vi "trigger-test3.vi"() -> ()   [LabVIEW 2020]
uses:
  Realization/PI650 VoltageAmp/TypeDefs/Channel gain.ctl
  Realization/PIPX40 Matrix/PIPX40 Matrix.lvclass
  Realization/PI650 VoltageAmp/PI650 VoltageAmp.lvclass
  Realization/PI650 VoltageAmp/TypeDefs/Channel DC offset.ctl
  Realization/NI PXI Trigger/NI PXI Trigger.lvclass
  Realization/NI PXI Trigger/PXI Trigger config.ctl
  Realization/NI DMM/NI DMM.lvclass
  Realization/NI DMM/TypeDefs/DMM waveform settings.ctl
  <instrlib>/niDMM/nidmm.llb/niDMM Waveform Function.ctl
  Realization/NI DMM/TypeDefs/Trigger settings.ctl
  <instrlib>/niDMM/nidmm.llb/niDMM Trigger.ctl
  <instrlib>/niDMM/nidmm.llb/niDMM Slope.ctl
  Realization/NI Analog Input/NI Analog Input.lvclass
  Realization/NI DAQmx Base/TypeDefs/Channel Config.ctl
  Realization/NI Analog Output/TypeDefs/Trigger Config.ctl
  Realization/NI Analog Output/NI Analog Output.lvclass
  Realization/NI Analog Output/TypeDefs/Timing Config.ctl
  <vilib>/measure/NI_MABase.lvlib
panel:
  in  "noise level":dbl=0.05 format="%#_3f"
  in  "signal type":T1(ring)
  in  "Channel gain":T2={"Channel (CH1)"=3, "Gain (x1)"=2} {"Channel (CH1)" items=["CH1"=1, "CH2"=2, "CH3"=3, "CH4"=4, "CH5"=5]; "Gain (x1)" items=["x1"=1, "x2"=2, "x5"=3, "x7"=4, "x10"=5, "x14"=6, "x20"=7]}
  out "Amp Info":variant
  out "Mx infos":variant[](array[variant])
  out "Waveform Graph":dynamicdata(graph)
  out "error out":errorcluster
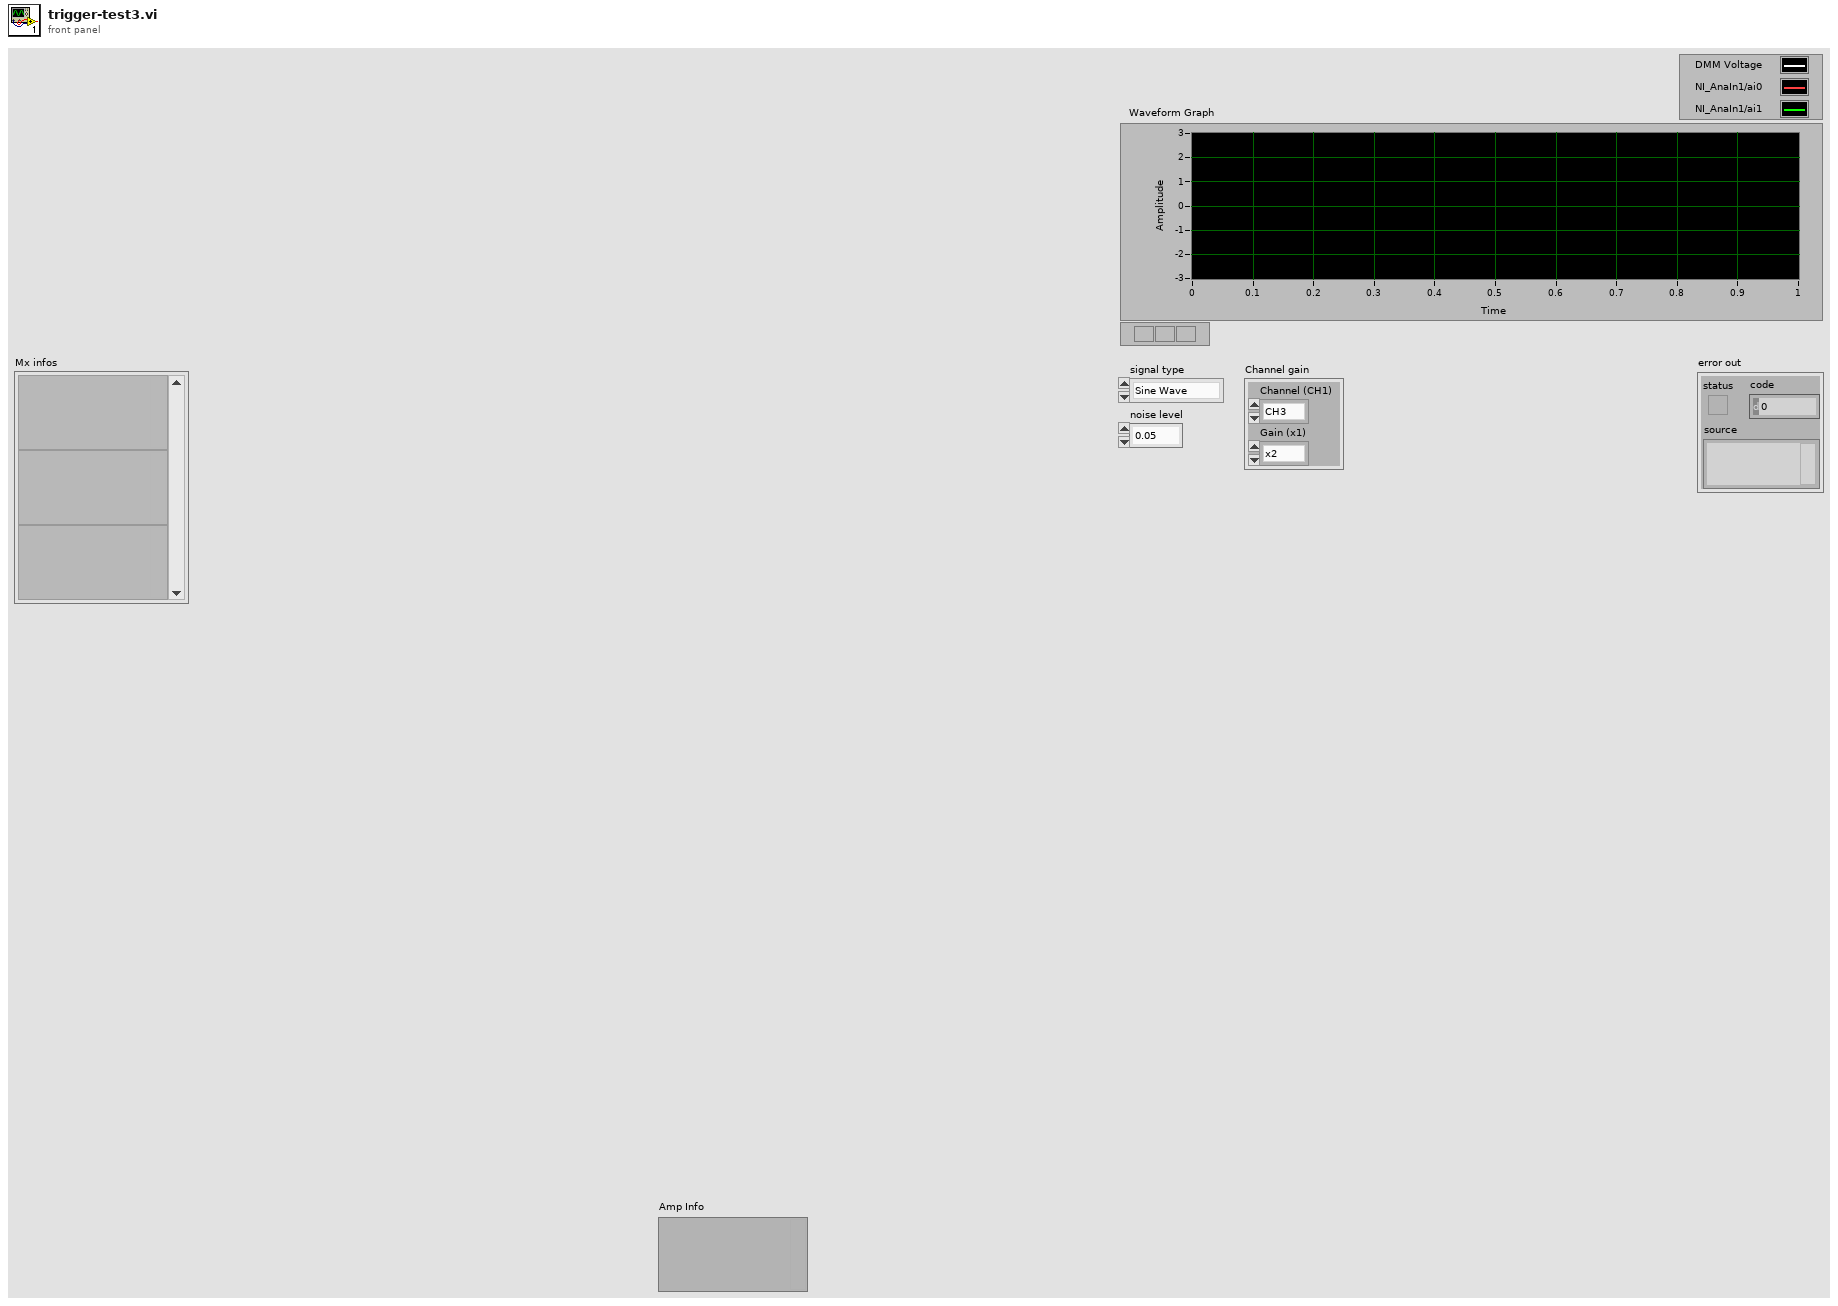
[diagram p1: front panel]
types:
  T1 = enum16{"Sine Wave", "Triangle Wave", "Square Wave", "Sawtooth Wave"}
  T2 = typedef "Channel gain.ctl" = cluster{"Channel (CH1)":u32, "Gain (x1)":u32}
  T3 = typedef "Trigger Config.ctl" = cluster{"trigger type":string, "source":string, "slope":i32, "analog level":dbl, "analog hysteresis":dbl}
  T4 = typedef "Timing Config.ctl" = cluster{"sample mode":i32, "samples per channel":i32, "rate":dbl, "source":string, "active edge":i32}
  T5 = typedef "Channel Config.ctl" = cluster{"channels":string, "maximum value":dbl, "minimum value":dbl, "output terminal configuration":i32, "units":i32}
  T6 = typedef "Trigger settings.ctl" = cluster{"Trigger Source":T7, "Trigger Delay (sec)":dbl, "Slope":T8}
  T7 = typedef "niDMM Trigger.ctl" = enum16{"Immediate", "External", "TTL 0", "TTL 1", "TTL 2", "TTL 3", "TTL 4", "TTL 5", "TTL 6", "Software", "TTL 7", "PXI Star", "LBR Trig 1", "Aux Trig 1"}
  T8 = typedef "niDMM Slope.ctl" = enum16{"Rising Edge", "Falling Edge"}
  T9 = typedef "DMM waveform settings.ctl" = cluster{"Waveform Points":i32, "Function":T10, "Rate":dbl, "Range":dbl, "\nSettle Time":dbl}
  T10 = typedef "niDMM Waveform Function.ctl" = i32
  T11 = typedef "PXI Trigger config.ctl" = cluster{"counter output":string, "source terminal":string, "destination terminal":string}
  T12 = typedef "Channel DC offset.ctl" = cluster{"Channel (CH1)":u32, "Offset (128)":u32}
  T13 = map{string, refnum<class "PIPX40 Matrix.lvclass">}
  T14 = cluster{"samples per channel":dbl, "samples per channel":dbl}
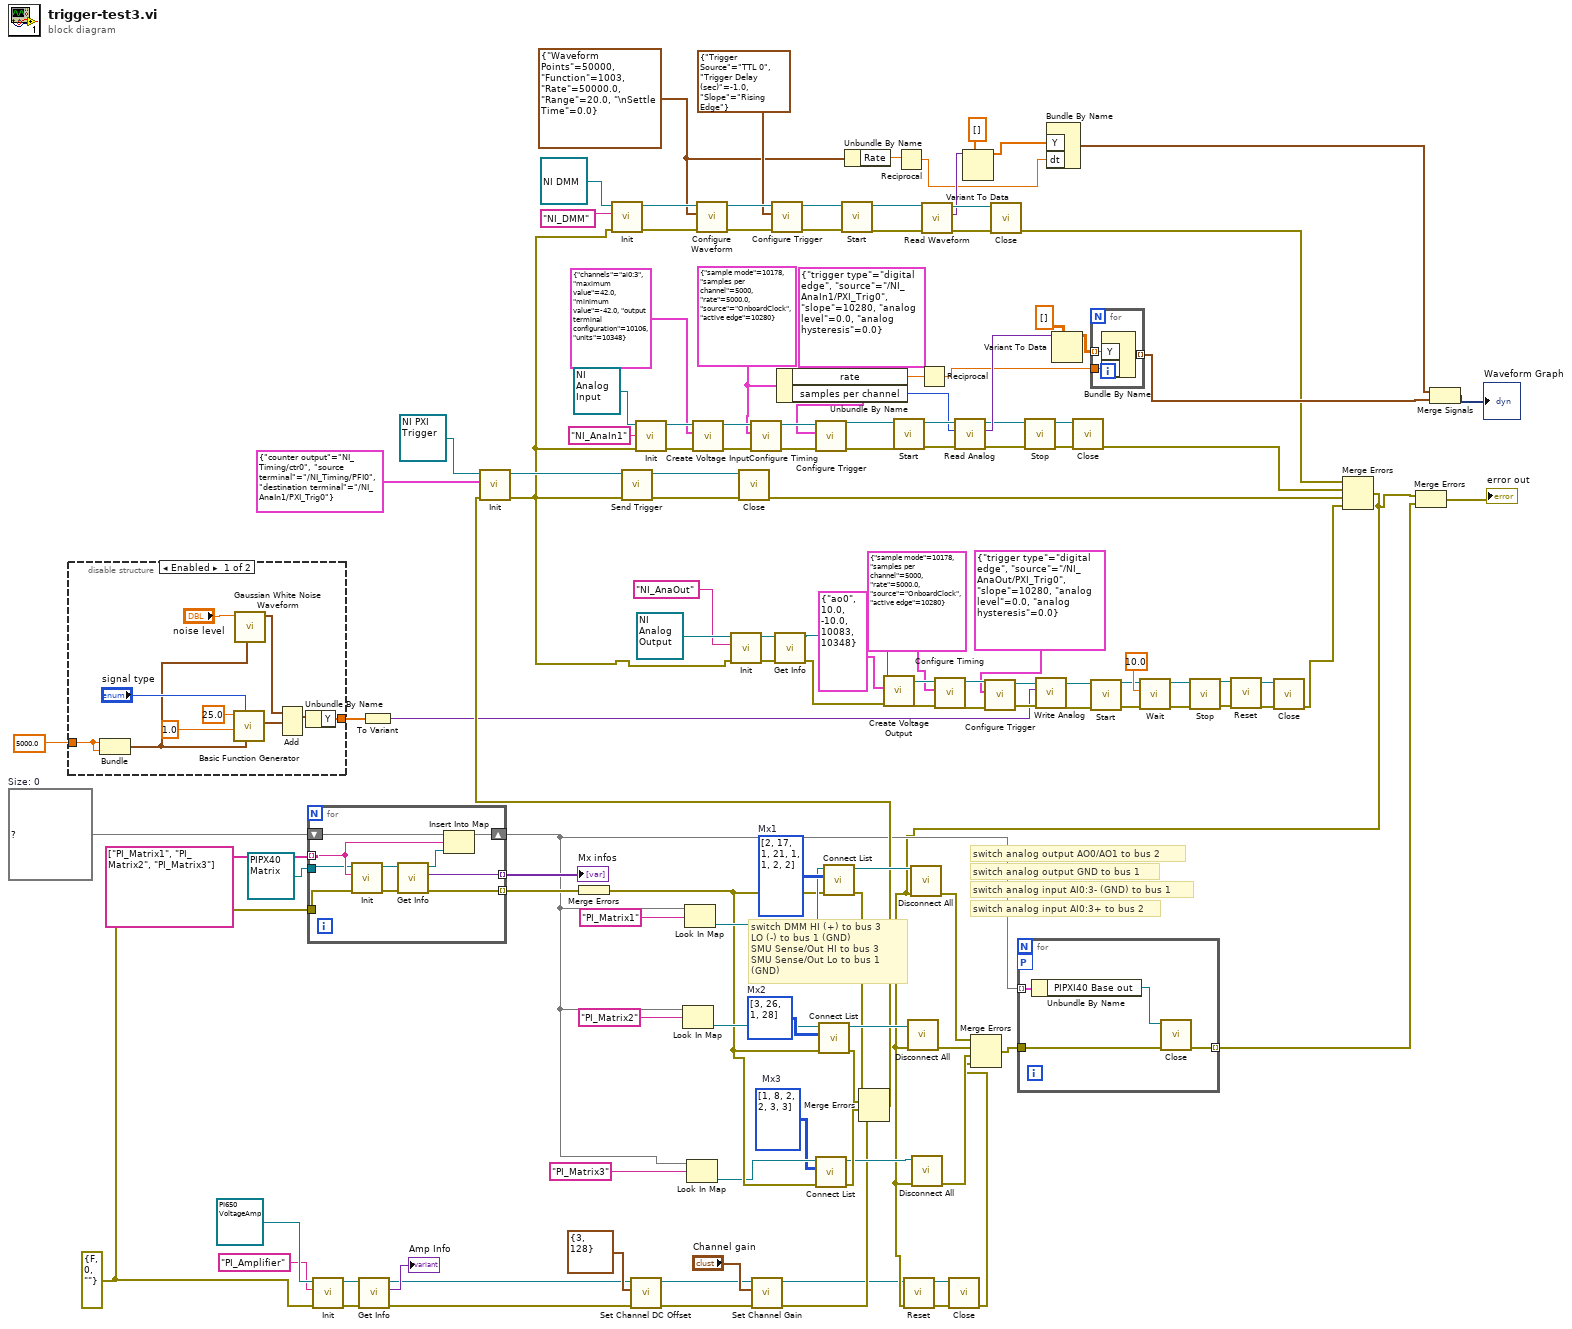
[diagram p0: block diagram]
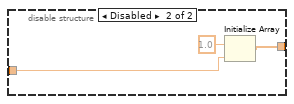
[diagram p2: hidden frame]
diagram:
  w32 = T4 {"sample mode"=10178, "samples per channel"=5000, "rate"=5000.0, "source"="OnboardClock", "active edge"=10280}
  w60 = T9 {"Waveform Points"=50000, "Function"=1003, "Rate"=50000.0, "Range"=20.0, "\nSettle Time"=0.0}
  w94 = errorcluster {"status"=FALSE, "code"=0, "source"=""} ("error in (no error)")
  w105 = i32[][] [[1, 8], [2, 2], [3, 3]]  # Mx3
  w116 = T13 {}  # Size: 0
  w125 = i32[][] [[3, 26], [1, 28]]  # Mx2
  w127 = i32[][] [[2, 17], [1, 21], [1, 1], [2, 2]]  # Mx1
  # "switch analog input AI0:3+ to bus 2"
  # "switch analog input AI0:3- (GND) to bus 1"
  # "switch analog output GND to bus 1"
  # "switch analog output AO0/AO1 to bus 2"
  # "switch DMM HI (+) to bus 3 \nLO (-) to bus 1 (GND)\nSMU Sense/Out HI to bus 3\nSMU Sense/Out Lo to bus 1 (GND)"
  n1 = disable-structure shown="Enabled" {
    disable-tunnel: 5000.0 ("samples per channel") -> [w141 w144]
    disable-tunnel: [w140 w146] -> w83
    frame Enabled {
      n2 = Bundle("samples per channel"=w141, "samples per channel"=w141) -> (w138:T14)  [unwired: 1 in]
      n3 = call <vilib>:"Basic Function Generator.vi"("sampling info"=w138, "signal type"="signal type", "amplitude"=1.0, "frequency"=25.0) -> ("signal out"=w137:waveform(dbl))  [unwired: 5 in, 2 out]
      n4 = call <vilib>:"Gaussian White Noise Waveform.vi"("sampling info"=w138, "standard deviation"="noise level") -> ("signal out"=w136:waveform(dbl))  [unwired: 8 in, 1 out]
      n5 = Add(1:w137, 2:w136) -> (0:w135:waveform(dbl))  [unwired: 1 in, 1 out]
      n6 = Unbundle By Name(w135) -> ("Y"=w140:dbl[])
    }
    frame Disabled {
      n7 = Initialize Array(1.0 ("element"), w144) -> (w146:dbl[])
    }
  }
  n8 = for {
    tunnel: string[] ["PI_Matrix1", "PI_Matrix2", "PI_Matrix3"] -> [w152] mode=indexing
    tunnel: [w155] -> w130 mode=indexing
    tunnel: [w154] -> w129 mode=indexing
    shift-right: [w153] -> w108
    shift-left: w116 -> [w150]
    tunnel: refnum<class "PIPX40 Matrix.lvclass"> refnum ("PIPXI40 Matrix in") -> [w148]
    tunnel: w94 -> [w147]
    n9 = call-dynamic "Init.vi"("error in (no error)"=w147, "Params"=w152, "PIPXI40 Base in"=w148) -> ("error out"=w156:errorcluster, "PIPXI40 Base out"=w151:refnum<class "PIPX40 Matrix.lvclass">)  [unwired: 7 in]
    n10 = call-dynamic "Get Info.vi"("error in (no error)"=w156, "PIPXI40 Base in"=w151) -> ("error out"=w155:errorcluster, "Info"=w154:variant, "PIPXI40 Base out"=w149:refnum<class "PIPX40 Matrix.lvclass">)  [unwired: 7 in]
    n11 = Insert Into Map(map in=w150, key=w152, value=w149) -> (map out=w153:T13)  [unwired: 2 out]
  }
  "Mx infos" <- w129
  n12 = call-dynamic "Init.vi"("error in (no error)"=w94, "Params"="PI_Amplifier" ("String"), "PI650 VoltageAmp in"=refnum<class "PI650 VoltageAmp.lvclass"> refnum) -> ("error out"=w99:errorcluster, "PI650 VoltageAmp out"=w100:refnum<class "PI650 VoltageAmp.lvclass">)  [unwired: 7 in]
  n13 = call-dynamic "Get Info.vi"("error in (no error)"=w99, "PI650 VoltageAmp in"=w100) -> ("error out"=w93:errorcluster, "Info"=→"Amp Info":variant, "PI650 VoltageAmp out"=w92:refnum<class "PI650 VoltageAmp.lvclass">)  [unwired: 7 in]
  n14 = To Variant(anything=w83) -> (Variant=w1:variant)
  n15 = Merge Errors(w130) -> (w107:errorcluster)
  n16 = call-dynamic "Set Channel DC Offset.vi"("error in (no error)"=w93, "Params"=T12 {"Channel (CH1)"=3, "Offset (128)"=128}, "PI650 VoltageAmp in"=w92) -> ("error out"=w90:errorcluster, "PI650 VoltageAmp out"=w91:refnum<class "PI650 VoltageAmp.lvclass">)  [unwired: 7 in]
  n17 = Look In Map(map=w108, key="PI_Matrix2" ("String")) -> (value=w118:refnum<class "PIPX40 Matrix.lvclass">)  [unwired: 1 in, 1 out]
  n18 = Look In Map(map=w108, key="PI_Matrix1" ("String")) -> (value=w119:refnum<class "PIPX40 Matrix.lvclass">)  [unwired: 1 in, 1 out]
  n19 = Look In Map(map=w108, key="PI_Matrix3" ("String")) -> (value=w106:refnum<class "PIPX40 Matrix.lvclass">)  [unwired: 1 in, 1 out]
  n20 = call-dynamic "Set Channel Gain.vi"("error in (no error)"=w90, "Params"="Channel gain", "PI650 VoltageAmp in"=w91) -> ("error out"=w89:errorcluster, "PI650 VoltageAmp out"=w85:refnum<class "PI650 VoltageAmp.lvclass">)  [unwired: 7 in]
  n21 = Unbundle By Name(w32) -> ("rate"=w30:dbl, "samples per channel"=w31:i32)
  n22 = call-dynamic "Connect List.vi"("error in (no error)"=w107, "Params"=w105, "PIPXI40 Matrix in"=w106) -> ("error out"=w104:errorcluster, "PIPXI40 Matrix out"=w103:refnum<class "PIPX40 Matrix.lvclass">)  [unwired: 7 in]
  n23 = call-dynamic "Connect List.vi"("error in (no error)"=w107, "Params"=w125, "PIPXI40 Matrix in"=w118) -> ("error out"=w114:errorcluster, "PIPXI40 Matrix out"=w123:refnum<class "PIPX40 Matrix.lvclass">)  [unwired: 7 in]
  n24 = call-dynamic "Connect List.vi"("error in (no error)"=w107, "Params"=w127, "PIPXI40 Matrix in"=w119) -> ("error out"=w115:errorcluster, "PIPXI40 Matrix out"=w124:refnum<class "PIPX40 Matrix.lvclass">)  [unwired: 7 in]
  n25 = Unbundle By Name(w60) -> ("Rate"=w59:dbl)
  n26 = Merge Errors(w115, w114, w104, w89) -> (w113:errorcluster)
  n27 = call-dynamic "Init.vi"("error in (no error)"=w113, "Params"=T11 {"counter output"="NI_Timing/ctr0", "source terminal"="/NI_Timing/PFI0", "destination terminal"="/NI_AnaIn1/PXI_Trig0"} ("Cluster of class private data"), "NI PXI Trigger in"=refnum<class "NI PXI Trigger.lvclass"> refnum) -> ("error out"=w2:errorcluster, "NI PXI Trigger out"=w80:refnum<class "NI PXI Trigger.lvclass">)  [unwired: 7 in]
  n28 = call-dynamic "Init.vi"("error in (no error)"=w2, "Params"="NI_DMM", "NI DMM in"=refnum<class "NI DMM.lvclass"> refnum) -> ("error out"=w75:errorcluster, "NI DMM out"=w76:refnum<class "NI DMM.lvclass">)  [unwired: 7 in]
  n29 = call-dynamic "Send Trigger.vi"("error in (no error)"=w2, "NI PXI Trigger in"=w80) -> ("error out"=w79:errorcluster, "NI PXI Trigger out"=w78:refnum<class "NI PXI Trigger.lvclass">)  [unwired: 8 in]
  n30 = call-dynamic "Init.vi"("error in (no error)"=w2, "Params"="NI_AnaIn1" ("String"), "DAQmx Base in"=refnum<class "NI Analog Input.lvclass"> refnum ("NI Analog Input in")) -> ("error out"=w52:errorcluster, "DAQmx Base out"=w51:refnum<class "NI Analog Input.lvclass">)  [unwired: 7 in]
  n31 = call-dynamic "Create Voltage Input.vi"("error in (no error)"=w52, "Params"=T5 {"channels"="ai0:3", "maximum value"=42.0, "minimum value"=-42.0, "output terminal configuration"=10106, "units"=10348} ("Channel Config"), "NI Analog Input in"=w51) -> ("error out"=w53:errorcluster, "NI Analog Input out"=w50:refnum<class "NI Analog Input.lvclass">)  [unwired: 7 in]
  n32 = call-dynamic "Configure Waveform.vi"("error in (no error)"=w75, "Params"=w60, "NI DMM in"=w76) -> ("error out"=w71:errorcluster, "NI DMM out"=w72:refnum<class "NI DMM.lvclass">)  [unwired: 7 in]
  n33 = call-dynamic "Init.vi"("error in (no error)"=w2, "Params"="NI_AnaOut" ("String"), "DAQmx Base in"=refnum<class "NI Analog Output.lvclass"> refnum ("NI DAQmx.lvlib:NI Analog Output.lvclass")) -> ("error out"=w26:errorcluster, "DAQmx Base out"=w27:refnum<class "NI Analog Output.lvclass">)  [unwired: 7 in]
  n34 = call-dynamic "Close.vi"("error in (no error)"=w79, "NI PXI Trigger in"=w78) -> ("error out"=w56:errorcluster)  [unwired: 8 in, 1 out]
  n35 = call-dynamic "Configure Timing.vi"("error in (no error)"=w53, "Params"=w32, "NI DAQmx Base in"=w50) -> ("error out"=w48:errorcluster, "NI DAQmx Base out"=w49:refnum<class "NI Analog Input.lvclass">)  [unwired: 7 in]
  n36 = call-dynamic "Configure Trigger.vi"("error in (no error)"=w71, "Params"=T6 {"Trigger Source"=enum."TTL 0", "Trigger Delay (sec)"=-1.0, "Slope"=enum."Rising Edge"}, "NI DMM in"=w72) -> ("error out"=w69:errorcluster, "NI DMM out"=w70:refnum<class "NI DMM.lvclass">)  [unwired: 7 in]
  n37 = call-dynamic "Get Info.vi"("error in (no error)"=w26, "DAQmx Base in"=w27) -> ("error out"=w3:errorcluster, "DAQmx Base out"=w23:refnum<class "NI Analog Output.lvclass">)  [unwired: 7 in, 1 out]
  n38 = call-dynamic "Configure Trigger.vi"("error in (no error)"=w48, "Params"=T3 {"trigger type"="digital edge", "source"="/NI_AnaIn1/PXI_Trig0", "slope"=10280, "analog level"=0.0, "analog hysteresis"=0.0}, "NI DAQmx Base in"=w49) -> ("error out"=w42:errorcluster, "NI DAQmx Base out"=w41:refnum<class "NI Analog Input.lvclass">)  [unwired: 7 in]
  n39 = call-dynamic "Start.vi"("error in (no error)"=w69, "DMM in"=w70) -> ("error out"=w67:errorcluster, "DMM out"=w68:refnum<class "NI DMM.lvclass">)  [unwired: 8 in]
  n40 = call-dynamic "Create Voltage Output.vi"("error in (no error)"=w3, "Params"=T5 {"channels"="ao0", "maximum value"=10.0, "minimum value"=-10.0, "output terminal configuration"=10083, "units"=10348} ("Channel Config"), "NI Analog Output in"=w23) -> ("error out"=w22:errorcluster, "NI Analog Output out"=w21:refnum<class "NI Analog Output.lvclass">)  [unwired: 7 in]
  n41 = call-dynamic "Start.vi"("error in (no error)"=w42, "NI DAQmx Base in"=w41) -> ("error out"=w43:errorcluster, "NI DAQmx Base out"=w40:refnum<class "NI Analog Input.lvclass">)  [unwired: 8 in]
  n42 = Reciprocal(x=w59) -> (1/x=w58:dbl)
  n43 = Reciprocal(x=w30) -> (1/x=w29:dbl)
  n44 = call-dynamic "Read Waveform.vi"("error in (no error)"=w67, "NI DMM in"=w68) -> ("error out"=w65:errorcluster, "Data"=w63:variant, "NI DMM out"=w64:refnum<class "NI DMM.lvclass">)  [unwired: 7 in]
  n45 = call-dynamic "Configure Timing.vi"("error in (no error)"=w22, "Params"=T4 {"sample mode"=10178, "samples per channel"=5000, "rate"=5000.0, "source"="OnboardClock", "active edge"=10280}, "NI DAQmx Base in"=w21) -> ("error out"=w8:errorcluster, "NI DAQmx Base out"=w7:refnum<class "NI Analog Output.lvclass">)  [unwired: 7 in]
  n46 = call-dynamic "Read Analog.vi"("error in (no error)"=w43, "Params"=w31, "NI Analog Input in"=w40) -> ("error out"=w35:errorcluster, "Data"=w38:variant, "NI Analog Input out"=w36:refnum<class "NI Analog Input.lvclass">)  [unwired: 6 in]
  n47 = Variant To Data(type=dbl[] [], Variant=w63) -> (data=w61:dbl[])  [unwired: 1 in, 1 out]
  n48 = call-dynamic "Configure Trigger.vi"("error in (no error)"=w8, "Params"=T3 {"trigger type"="digital edge", "source"="/NI_AnaOut/PXI_Trig0", "slope"=10280, "analog level"=0.0, "analog hysteresis"=0.0}, "NI DAQmx Base in"=w7) -> ("error out"=w5:errorcluster, "NI DAQmx Base out"=w6:refnum<class "NI Analog Output.lvclass">)  [unwired: 7 in]
  n49 = call-dynamic "Close.vi"("error in (no error)"=w65, "NI DMM in"=w64) -> ("error out"=w54:errorcluster)  [unwired: 8 in, 1 out]
  n50 = call-dynamic "Stop.vi"("error in (no error)"=w35, "NI DAQmx Base in"=w36) -> ("error out"=w34:errorcluster, "NI DAQmx Base out"=w37:refnum<class "NI Analog Input.lvclass">)  [unwired: 8 in]
  n51 = call-dynamic "Write Analog.vi"("error in (no error)"=w5, "Params"=w1, "NI Analog Output in"=w6) -> ("error out"=w19:errorcluster, "NI Analog Output out"=w18:refnum<class "NI Analog Output.lvclass">)  [unwired: 7 in]
  n52 = Bundle By Name("Y"=w61, "dt"=w58) -> (w57:waveform(dbl))  [unwired: 1 in]
  n53 = Variant To Data(type=dbl[][] [], Variant=w38) -> (data=w33:dbl[][])  [unwired: 1 in, 1 out]
  n54 = call-dynamic "Close.vi"("error in (no error)"=w34, "DAQmx Base in"=w37) -> ("error out"=w55:errorcluster)  [unwired: 8 in, 1 out]
  n55 = for {
    tunnel: w33 -> [w159] mode=indexing
    tunnel: [w158] -> w82 mode=indexing
    tunnel: w29 -> [w157]
    n56 = Bundle By Name("Y"=w159, "dt"=w157) -> (w158:waveform(dbl))  [unwired: 1 in]
  }
  n57 = call-dynamic "Start.vi"("error in (no error)"=w19, "NI DAQmx Base in"=w18) -> ("error out"=w12:errorcluster, "NI DAQmx Base out"=w11:refnum<class "NI Analog Output.lvclass">)  [unwired: 8 in]
  n58 = call-dynamic "Wait.vi"("error in (no error)"=w12, "Params"=10.0, "NI DAQmx Base in"=w11) -> ("error out"=w14:errorcluster, "NI DAQmx Base out"=w15:refnum<class "NI Analog Output.lvclass">)  [unwired: 7 in]
  n59 = call-dynamic "Stop.vi"("error in (no error)"=w14, "NI DAQmx Base in"=w15) -> ("error out"=w17:errorcluster, "NI DAQmx Base out"=w16:refnum<class "NI Analog Output.lvclass">)  [unwired: 8 in]
  n60 = call-dynamic "Reset.vi"("error in (no error)"=w17, "DAQmx Base in"=w16) -> ("error out"=w10:errorcluster, "DAQmx Base out"=w9:refnum<class "NI Analog Output.lvclass">)  [unwired: 8 in]
  n61 = call-dynamic "Close.vi"("error in (no error)"=w10, "DAQmx Base in"=w9) -> ("error out"=w132:errorcluster)  [unwired: 8 in, 1 out]
  n62 = Merge Errors(w54, w55, w56, w132) -> (w86:errorcluster)
  n63 = call-dynamic "Reset.vi"("error in (no error)"=w86, "PI650 VoltageAmp in"=w85) -> ("error out"=w87:errorcluster, "PI650 VoltageAmp out"=w88:refnum<class "PI650 VoltageAmp.lvclass">)  [unwired: 8 in]
  n64 = call-dynamic "Disconnect All.vi"("error in (no error)"=w86, "PIPXI40 Matrix in"=w123) -> ("error out"=w122:errorcluster)  [unwired: 8 in, 1 out]
  n65 = call-dynamic "Disconnect All.vi"("error in (no error)"=w86, "PIPXI40 Matrix in"=w124) -> ("error out"=w121:errorcluster)  [unwired: 8 in, 1 out]
  n66 = call-dynamic "Disconnect All.vi"("error in (no error)"=w86, "PIPXI40 Matrix in"=w103) -> ("error out"=w102:errorcluster)  [unwired: 8 in, 1 out]
  n67 = call-dynamic "Close.vi"("error in (no error)"=w87, "PI650 VoltageAmp in"=w88) -> ("error out"=w84:errorcluster)  [unwired: 8 in, 1 out]
  n68 = Merge Errors(w121, w122, w102, w84) -> (w120:errorcluster)
  n69 = for {
    tunnel: w120 -> [w162]
    tunnel: [w163] -> w112 mode=indexing
    workers-P: _ -> [_]
    tunnel: w108 -> [w161] mode=indexing
    n70 = Unbundle By Name(w161) -> ("PIPXI40 Base out"=w160:refnum<class "PIPX40 Matrix.lvclass">)
    n71 = call-dynamic "Close.vi"("error in (no error)"=w162, "PIPXI40 Base in"=w160) -> ("error out"=w163:errorcluster)  [unwired: 8 in, 1 out]
  }
  n72 = Merge Errors(w86, w112) -> (→"error out":errorcluster)
  n73 = Merge Signals(w57, w82) -> (→"Waveform Graph":dynamicdata)
